vi "Create TreeNodeBox.vi"(1 "Pmin":sgl[](array[numeric]), 2 "Pmax":sgl[](array[numeric]), 3 "Parent":i32=-1, 4 "Level":i32=-1) -> (0 "Box":T1={"Face 0"={"V0"=[], "V1"=[], "V2"=[], "V3"=[], "E0"=[], "E1"=[], "E2"=[], "E3"=[], "n^"=[], "Plane"=enum."XY"}, "Face 1"={"V0"=[], "V1"=[], "V2"=[], "V3"=[], "E0"=[], "E1"=[], "E2"=[], "E3"=[], "n^"=[], "Plane"=enum."XY"}, "Face 2"={"V0"=[], "V1"=[], "V2"=[], "V3"=[], "E0"=[], "E1"=[], "E2"=[], "E3"=[], "n^"=[], "Plane"=enum."XY"}, "Face 3"={"V0"=[], "V1"=[], "V2"=[], "V3"=[], "E0"=[], "E1"=[], "E2"=[], "E3"=[], "n^"=[], "Plane"=enum."XY"}, "Face 4"={"V0"=[], "V1"=[], "V2"=[], "V3"=[], "E0"=[], "E1"=[], "E2"=[], "E3"=[], "n^"=[], "Plane"=enum."XY"}, "Face 5"={"V0"=[], "V1"=[], "V2"=[], "V3"=[], "E0"=[], "E1"=[], "E2"=[], "E3"=[], "n^"=[], "Plane"=enum."XY"}, "Level"=-1, "Pmax"=[], "Pmin"=[], "Parent"=-1, "Child 1"=-1, "Child 2"=-1, "Child 3"=-1, "Child 4"=-1, "Child 5"=-1, "Child 6"=-1, "Child 7"=-1, "Child 8"=-1, "Triangles"=[], "is leaf node"=FALSE})   [LabVIEW 2014]
uses:
  Typedefs/TreeNodeBox.ctl
  Typedefs/Quad.ctl
  Typedefs/Quadplane enum.ctl
panel:
  # "PN 17/01/2015"
  # "Vertices"
  # "Edges"
  # "Unit normal"
  # "Plane ident."
  # "Vertices"
  # "Edges"
  # "Unit normal"
  # "Plane ident."
  # "Vertices"
  # "Edges"
  # "Unit normal"
  # "Plane ident."
  # "Vertices"
  # "Edges"
  # "Unit normal"
  # "Plane ident."
  # "Vertices"
  # "Edges"
  # "Unit normal"
  # "Plane ident."
  # "Vertices"
  # "Edges"
  # "Unit normal"
  # "Plane ident."
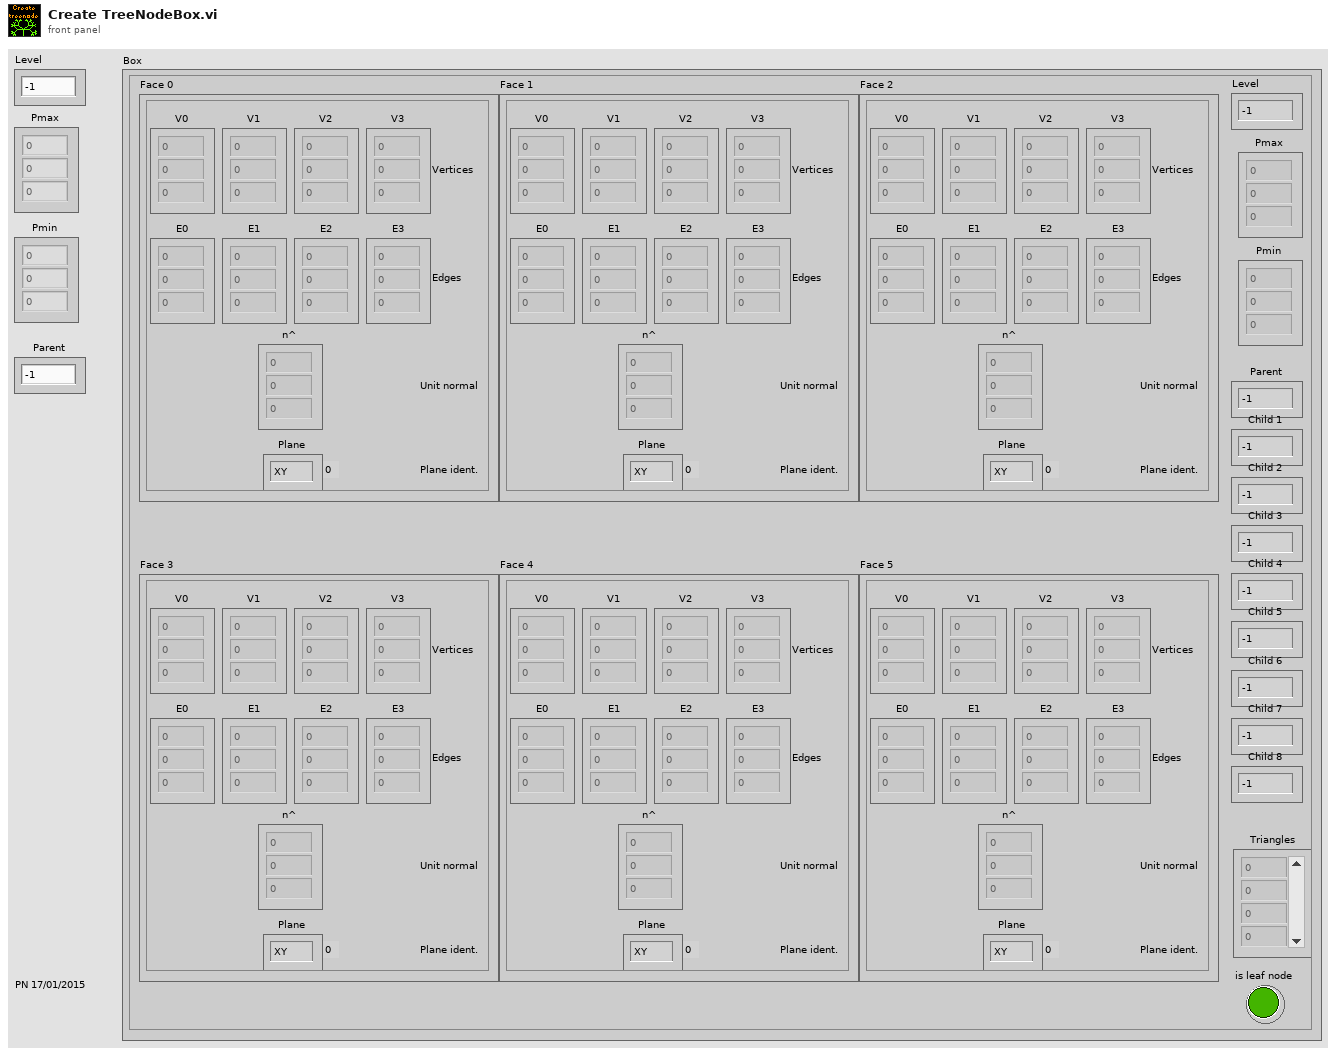
[diagram p1: front panel]
types:
  T1 = typedef "TreeNodeBox.ctl" = cluster{"Face 0":T2, "Face 1":T2, "Face 2":T2, "Face 3":T2, "Face 4":T2, "Face 5":T2, "Level":i32, "Pmax":sgl[], "Pmin":sgl[], "Parent":i32, "Child 1":i32, "Child 2":i32, "Child 3":i32, "Child 4":i32, "Child 5":i32, "Child 6":i32, "Child 7":i32, "Child 8":i32, "Triangles":i32[], "is leaf node":bool}
  T2 = typedef "Quad.ctl" = cluster{"V0":sgl[], "V1":sgl[], "V2":sgl[], "V3":sgl[], "E0":sgl[], "E1":sgl[], "E2":sgl[], "E3":sgl[], "n^":sgl[], "Plane":T3}
  T3 = typedef "Quadplane enum.ctl" = enum8{"XY", "XZ", "YZ", "-XY", "-XZ", "-YZ"}
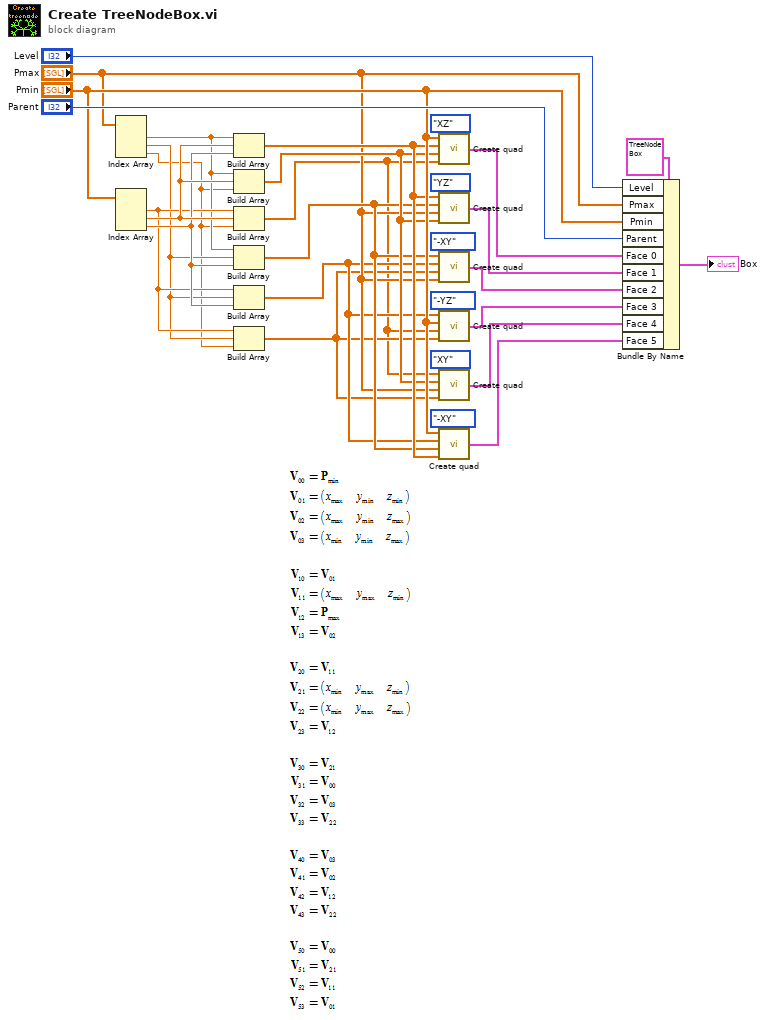
[diagram p0: block diagram]
diagram:
  n1 = Index Array(array="Pmax") -> (element #1=w11:sgl, element #2=w12:sgl, element #3=w7:sgl)  [unwired: 3 in]
  n2 = Index Array(array="Pmin") -> (element #1=w13:sgl, element #2=w18:sgl, element #3=w15:sgl)  [unwired: 3 in]
  n3 = Build Array(w11, w18, w15) -> (w20:sgl[])
  n4 = Build Array(w11, w18, w7) -> (w19:sgl[])
  n5 = Build Array(w13, w18, w7) -> (w9:sgl[])
  n6 = Build Array(w11, w12, w15) -> (w17:sgl[])
  n7 = Build Array(w13, w12, w15) -> (w14:sgl[])
  n8 = Build Array(w13, w12, w7) -> (w10:sgl[])
  n9 = call "Create quad.vi"("V0"="Pmin", "V1"=w20, "V2"=w19, "V3"=w9, "Plane"=Quadplane_enum."XZ") -> ("Quad"=w30:T2)
  n10 = call "Create quad.vi"("V0"=w20, "V1"=w17, "V2"="Pmax", "V3"=w19, "Plane"=Quadplane_enum."YZ") -> ("Quad"=w29:T2)
  n11 = call "Create quad.vi"("V0"=w17, "V1"=w14, "V2"=w10, "V3"="Pmax", "Plane"=Quadplane_enum."-XY") -> ("Quad"=w28:T2)
  n12 = call "Create quad.vi"("V0"=w14, "V1"="Pmin", "V2"=w9, "V3"=w10, "Plane"=Quadplane_enum."-YZ") -> ("Quad"=w27:T2)
  n13 = call "Create quad.vi"("V0"=w9, "V1"=w19, "V2"="Pmax", "V3"=w10, "Plane"=Quadplane_enum."XY") -> ("Quad"=w26:T2)
  n14 = call "Create quad.vi"("V0"="Pmin", "V1"=w14, "V2"=w17, "V3"=w20, "Plane"=Quadplane_enum."-XY") -> ("Quad"=w25:T2)
  n15 = Bundle By Name(cluster=T1 {"Face 0"={"V0"=[], "V1"=[], "V2"=[], "V3"=[], "E0"=[], "E1"=[], "E2"=[], "E3"=[], "n^"=[], "Plane"=enum."XY"}, "Face 1"={"V0"=[], "V1"=[], "V2"=[], "V3"=[], "E0"=[], "E1"=[], "E2"=[], "E3"=[], "n^"=[], "Plane"=enum."XY"}, "Face 2"={"V0"=[], "V1"=[], "V2"=[], "V3"=[], "E0"=[], "E1"=[], "E2"=[], "E3"=[], "n^"=[], "Plane"=enum."XY"}, "Face 3"={"V0"=[], "V1"=[], "V2"=[], "V3"=[], "E0"=[], "E1"=[], "E2"=[], "E3"=[], "n^"=[], "Plane"=enum."XY"}, "Face 4"={"V0"=[], "V1"=[], "V2"=[], "V3"=[], "E0"=[], "E1"=[], "E2"=[], "E3"=[], "n^"=[], "Plane"=enum."XY"}, "Face 5"={"V0"=[], "V1"=[], "V2"=[], "V3"=[], "E0"=[], "E1"=[], "E2"=[], "E3"=[], "n^"=[], "Plane"=enum."XY"}, "Level"=-1, "Pmax"=[], "Pmin"=[], "Parent"=-1, "Child 1"=-1, "Child 2"=-1, "Child 3"=-1, "Child 4"=-1, "Child 5"=-1, "Child 6"=-1, "Child 7"=-1, "Child 8"=-1, "Triangles"=[], "is leaf node"=FALSE} ("Box"), "Level"="Level", "Pmax"="Pmax", "Pmin"="Pmin", "Parent"="Parent", "Face 0"=w30, "Face 1"=w29, "Face 2"=w28, "Face 3"=w27, "Face 4"=w26, "Face 5"=w25) -> (→"Box":T1)
